vi "Demo1.vi"() -> ()   [LabVIEW 2014, in "SJ-210.lvlib" / "SJ-210.lvclass"]
uses:
  SJ-210Class/SJ-210.lvclass
  API/Typedef/ACQ Data.ctl
  DriverMasterAsync/builds/DriverMasterAsync.lvlibp/Modules/HAL/DriverMasterAsync/DriverMasterAsyncClass/DriverMasterAsync.lvclass
  API/SJ-210 Lib.lvlib
panel:
  out "ACQ Data":T1
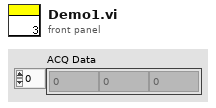
[diagram p1: front panel]
types:
  T1 = typedef "SJ-210 Lib.lvlib/ACQ Data.ctl" = sgl[]
  T2 = typedef "DriverMasterAsync.lvlibp/WINFAS 2 Data Queue.lvlib/Async Acquisition Data Cluster.ctl" = cluster{"Data":sgl[]}
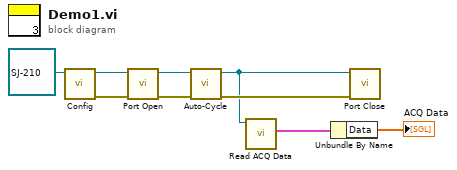
[diagram p0: block diagram]
diagram:
  n1 = call-dynamic "Config.vi"("SJ-210 in"=refnum<class "SJ-210.lvclass"> refnum) -> ("error out"=w7:errorcluster, "SJ-210 out"=w9:refnum<class "SJ-210.lvclass">)  [unwired: 9 in]
  n2 = call-dynamic "Port Open.vi"("error in (no error)"=w7, "SJ-210 in"=w9) -> ("error out"=w6:errorcluster, "SJ-210 out"=w8:refnum<class "SJ-210.lvclass">)  [unwired: 8 in]
  n3 = call-dynamic "Auto-Cycle.vi"("error in (no error)"=w6, "SJ-210 in"=w8) -> ("error out"=w5:errorcluster, "SJ-210 out"=w2:refnum<class "SJ-210.lvclass">)  [unwired: 8 in]
  n4 = call "Read ACQ Data.vi"("DriverMasterAsync in"=w2) -> ("ACQ Data"=w1:T2)  [unwired: 8 in, 2 out]
  n5 = Unbundle By Name(w1) -> ("Data"=→"ACQ Data":sgl[])
  n6 = call-dynamic "Port Close.vi"("error in (no error)"=w5, "SJ-210 in"=w2) -> ()  [unwired: 8 in, 2 out]
